vi "DAQ Error Manager.vi"(0 "Conductivity Error In":errorcluster, 1 "T1 Error In":errorcluster, 2 "T2 Error In":errorcluster, 3 "T3 Error In":errorcluster, 4 "T4 Error In":errorcluster, 5 "T5 Error In":errorcluster) -> (12 "Errors Present?":bool, 14 "Conductivity Error Out":errorcluster, 15 "T1 Error Out":errorcluster, 16 "T2 Error Out":errorcluster, 17 "T3 Error Out":errorcluster, 18 "T4 Error Out":errorcluster, 19 "T5 Error Out":errorcluster)   [LabVIEW 2016]
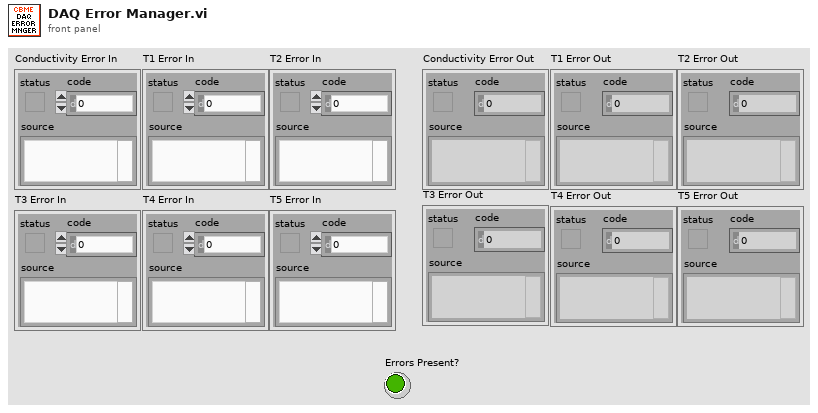
[diagram p1: front panel]
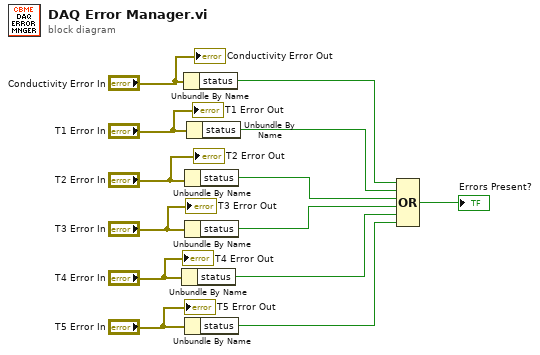
[diagram p0: block diagram]
diagram:
  n1 = Unbundle By Name("T4 Error In") -> ("status"=w3:bool)
  n2 = Unbundle By Name("Conductivity Error In") -> ("status"=w7:bool)
  n3 = Unbundle By Name("T2 Error In") -> ("status"=w5:bool)
  n4 = Unbundle By Name("T3 Error In") -> ("status"=w4:bool)
  n5 = Unbundle By Name("T5 Error In") -> ("status"=w2:bool)
  n6 = Unbundle By Name("T1 Error In") -> ("status"=w6:bool)
  n7 = Compound Arithmetic op=OR(w7, w6, w5, w4, w3, w2) -> (→"Errors Present?":bool)
  "Conductivity Error Out" <- "Conductivity Error In"
  "T1 Error Out" <- "T1 Error In"
  "T2 Error Out" <- "T2 Error In"
  "T3 Error Out" <- "T3 Error In"
  "T4 Error Out" <- "T4 Error In"
  "T5 Error Out" <- "T5 Error In"
